vi "Write IRQConfig.lvclass.vi"(8 "error in (no error)":errorcluster, 10 "IRQConfig.lvclass":refnum<class "IRQConfig.lvclass">, 11 "IRQHandler in":refnum<class "IRQHandler.lvclass">) -> (0 "error out":errorcluster, 3 "IRQHandler out":refnum<class "IRQHandler.lvclass">)   [LabVIEW 2013, in "ComponentData.lvlib" / "IRQHandler.lvclass"]
uses:
  <userlib>/Common/Component/common_application/RT/ComponentData/IRQHandler/IRQHandler.lvclass
  <userlib>/Common/Component/common_application/RT/ComponentData/ConfigurationHandler/IRQConfig/IRQConfig.lvclass
  <userlib>/Common/Component/common_application/RT/ComponentData/IRQHandler/IRQHandler.lvclass/IRQHandler.ctl
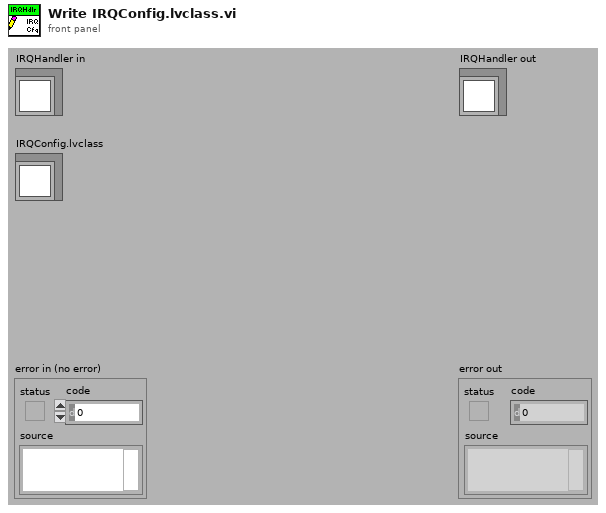
[diagram p1: front panel]
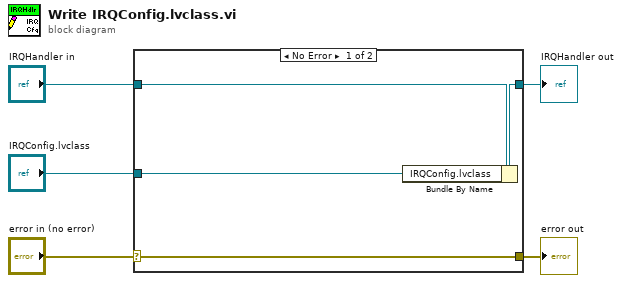
[diagram p0: block diagram]
diagram:
  n1 = case shown="No Error" "error in (no error)" {
    selector: "error in (no error)" -> [w9 w10]
    tunnel: [w9 w10] -> w4
    tunnel: [w7 w11] -> w2
    tunnel: "IRQHandler in" -> [w8 w11]
    tunnel: "IRQConfig.lvclass" -> [w6 _]
    frame No Error {
      n2 = Bundle By Name(cluster=w8, "IRQConfig.lvclass"=w6) -> (w7:refnum<class "IRQHandler.lvclass">)
    }
    frame Error {
    }
  }
  "error out" <- w4
  "IRQHandler out" <- w2
